vi "Init AI Resources.vi"(8 "error in (no error)":errorcluster, 11 "Session in":refnum<class "Session.lvclass">) -> (0 "error out":errorcluster, 3 "Session out":refnum<class "Session.lvclass">)   [LabVIEW 2020, in "CTI.lvlib" / "Session.lvclass"]
uses:
  Session.lvclass
  Session.lvclass/Session.ctl
  AI/AI.lvclass
  ADC Number.ctl
  CTI.lvlib
  DeviceComms/DeviceComms.lvclass
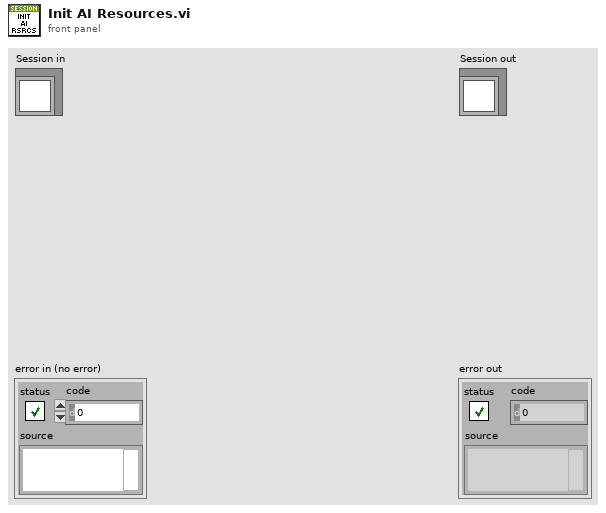
[diagram p1: front panel]
types:
  T1 = typedef "CTI.lvlib/ADC Number.ctl" = i8
  T2 = typedef "CTI.lvlib/Available AI.ctl" = cluster{"ADC #":T1, "GPIO #":T3}
  T3 = typedef "CTI.lvlib/GPIO Number.ctl" = i8
  T4 = typedef "CTI.lvlib/Session.lvclass/Resources.ctl" = cluster{"GPIO":map{T3, refnum<class "GPIO.lvclass">}, "AI":map{T1, refnum<class "AI.lvclass">}, "PWM":map{T3, refnum<class "PWM.lvclass">}, "UART":map{T5, refnum<class "UART.lvclass">}, "I2C":map{T6, refnum<class "I2C.lvclass">}, "SPI":map{T7, refnum<class "SPI.lvclass">}, "CS":map{T3, refnum<class "SPI CS.lvclass">}}
  T5 = typedef "CTI.lvlib/UART Number.ctl" = i8
  T6 = typedef "CTI.lvlib/I2C Number.ctl" = i8
  T7 = typedef "CTI.lvlib/SPI Number.ctl" = i8
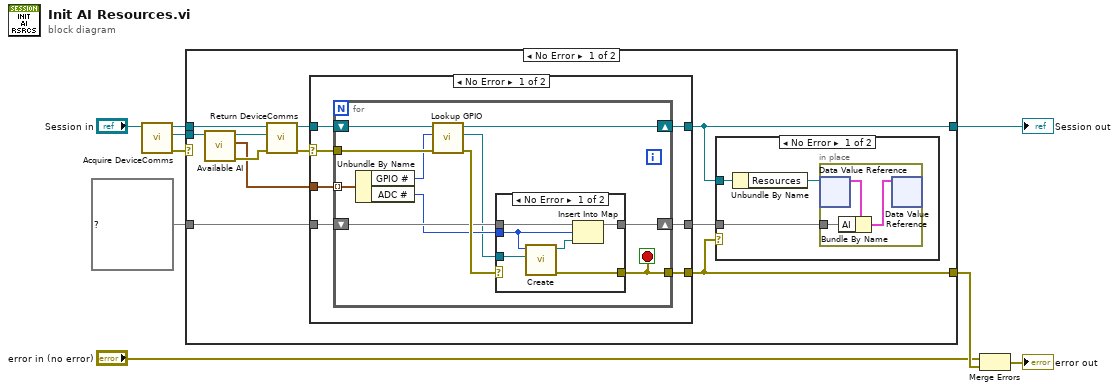
[diagram p0: block diagram]
diagram:
  n1 = call "Acquire DeviceComms.vi"("Session in"="Session in") -> ("error out"=w8:errorcluster, "DeviceComms"=w7:refnum<class "DeviceComms.lvclass">, "Session out"=w6:refnum<class "Session.lvclass">)  [unwired: 8 in]
  n2 = case shown="No Error" w8 {
    selector: w8 -> [_ w57]
    tunnel: w7 -> [w19 _]
    tunnel: w6 -> [w18 w56]
    tunnel: [w10 w56] -> w5
    tunnel: map{T1, refnum<class "AI.lvclass">} {} ("AI") -> [w14 _]
    tunnel: [w11 w57] -> w4
    frame No Error {
      n3 = call-dynamic "Available AI.vi"("DeviceComms in"=w19) -> ("error out"=w20:errorcluster, "Available AI"=w16:T2[], "DeviceComms out"=w17:refnum<class "DeviceComms.lvclass">)  [unwired: 8 in]
      n4 = call "Return DeviceComms.vi"("error in (no error)"=w20, "DeviceComms"=w17, "Session in"=w18) -> ("error out"=w12:errorcluster, "Session out"=w13:refnum<class "Session.lvclass">)  [unwired: 7 in]
      n5 = case shown="No Error" w12 {
        selector: w12 -> [w23 w49]
        tunnel: w16 -> [w27 _]
        tunnel: [w26 w47] -> w15
        tunnel: w14 -> [w25 w47]
        tunnel: w13 -> [w24 w48]
        tunnel: [w22 w48] -> w10
        tunnel: [w21 w49] -> w11
        frame No Error {
          n6 = for {
            tunnel: w27 -> [w34] mode=indexing
            shift-right: [w35] -> w26
            shift-left: w25 -> [w36]
            shift-right: [w30] -> w22
            shift-left: w24 -> [w33]
            tunnel: w23 -> [w38]
            tunnel: [w28] -> w21
            stop <- w28 stop-if-true
            n7 = Unbundle By Name(w34) -> ("GPIO #"=w32:T3, "ADC #"=w31:T1)
            n8 = call "Lookup GPIO.vi"("error in (no error)"=w38, "GPIO #"=w32, "Session in"=w33) -> ("error out"=w37:errorcluster, "GPIO"=w29:refnum<class "GPIO.lvclass">, "Session out"=w30:refnum<class "Session.lvclass">)  [unwired: 6 in]
            n9 = case shown="No Error" w37 {
              selector: w37 -> [_ w46]
              tunnel: w36 -> [w44 w45]
              tunnel: [w43 w45] -> w35
              tunnel: w29 -> [w42 _]
              tunnel: w31 -> [w41 _]
              tunnel: [w39 w46] -> w28
              frame No Error {
                n10 = call "Create.vi"("GPIO"=w42, "ADC #"=w41) -> ("error out"=w39:errorcluster, "AnalogIn out"=w40:refnum<class "AI.lvclass">)  [unwired: 8 in]
                n11 = Insert Into Map(map in=w44, key=w41, value=w40) -> (map out=w43:map{T1, refnum<class "AI.lvclass">})  [unwired: 2 out]
              }
              frame Error {
              }
            }
          }
        }
        frame Error {
        }
      }
      n12 = case shown="No Error" w11 {
        tunnel: w15 -> [w50 _]
        tunnel: w10 -> [w52 _]
        frame No Error {
          n13 = Unbundle By Name(w52) -> ("Resources"=w51:refnum<data-value>)
          n14 = in-place {
            in-place-border: w50 -> [w54]
            n15 = in-place-dvr #1(w51) -> (w55:T4)  [unwired: 1 out]
            n16 = Bundle By Name(cluster=w55, "AI"=w54) -> (w53:T4)
            n17 = in-place-dvr #1(w53) -> ()  [unwired: 2 out]
          }
        }
        frame Error {
        }
      }
    }
    frame Error {
    }
  }
  "Session out" <- w5
  n18 = Merge Errors("error in (no error)", w4) -> (→"error out":errorcluster)
